vi "Simple Actor Example.vi"() -> ()   [LabVIEW 2012]
uses:
  <vilib>/ActorFramework/Message Enqueuer/Message Enqueuer.lvclass
  <vilib>/ActorFramework/LastAck/Last Ack.lvclass
  <vilib>/ActorFramework/Message Queue/Message Queue.lvclass/Message Queue.ctl
  <vilib>/ActorFramework/Message Dequeuer/Message Dequeuer.lvclass/Message Dequeuer.ctl
  Simple Actor/Simple Actor.lvclass
  <vilib>/ActorFramework/LastAck/Last Ack.lvclass/Last Ack.ctl
  Simple Actor/Simple Actor.lvclass/Simple Actor.ctl
  <vilib>/ActorFramework/Message Enqueuer/Message Enqueuer.lvclass/Message Enqueuer.ctl
  <vilib>/ActorFramework/Message Enqueuer/Enqueue.vi
  <vilib>/ActorFramework/Message Priority Queue/Priority Dequeue.vi
  <vilib>/ActorFramework/Message Priority Queue/Priority Enqueue.vi
  <vilib>/ActorFramework/Stop Msg/Stop Msg.lvclass
  Simple Actor Messages/Zero Msg/Zero Msg.lvclass
  <vilib>/ActorFramework/Actor/Actor.lvclass
  <vilib>/ActorFramework/Message Queue/Message Queue.lvclass
  <vilib>/ActorFramework/Message Dequeuer/Message Dequeuer.lvclass
panel:
  in  "Target Actor":u16(ring) items=["0", "2"]
  in  "Synch":bool
  in  "Process Stop Button":bool
  in  "Refresh Button":bool
  in  "New Button":bool
  in  "stop":bool
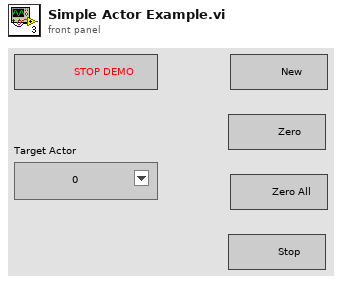
[diagram p1: front panel]
types:
  T1 = enum8{"Enabled", "Disabled", "Disabled and Grayed Out"}
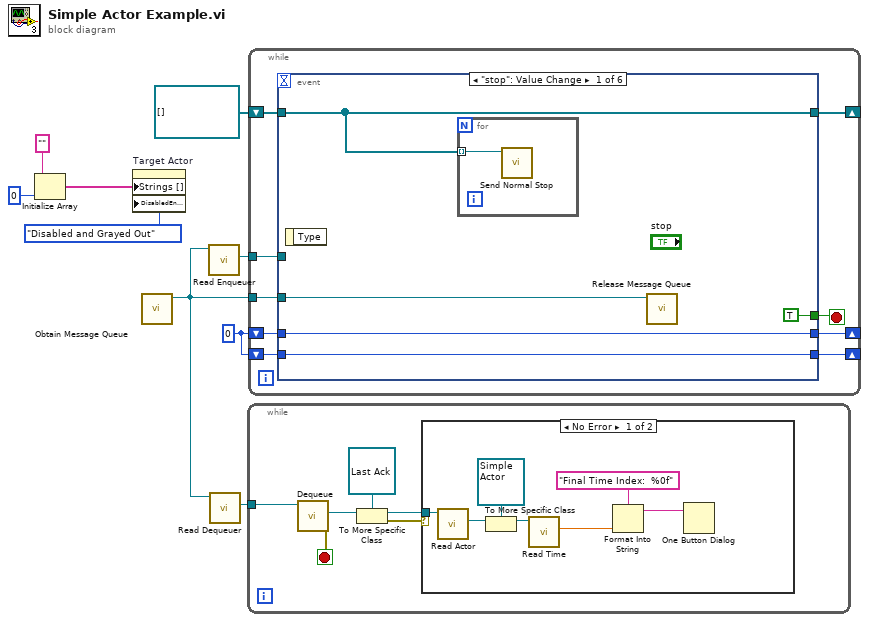
[diagram p0: block diagram]
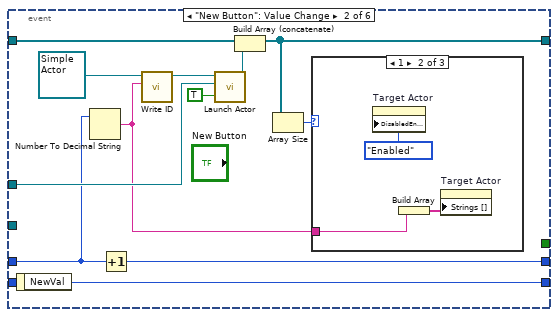
[diagram p3: hidden frame]
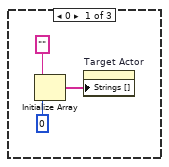
[diagram p4: hidden frame]
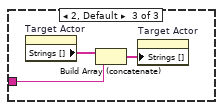
[diagram p5: hidden frame]
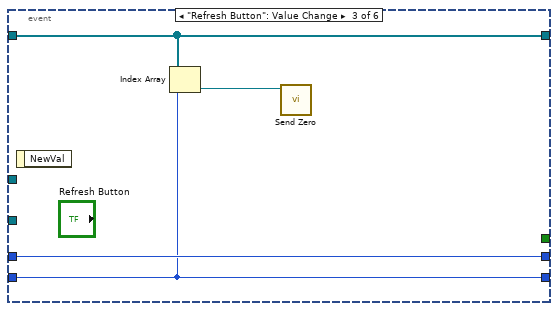
[diagram p6: hidden frame]
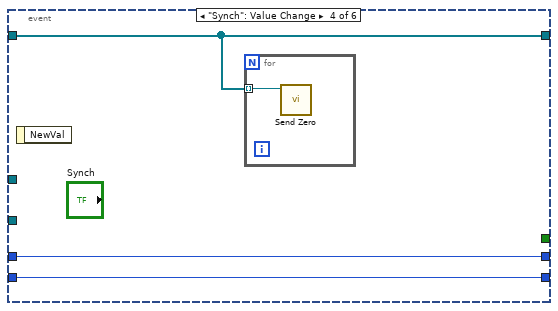
[diagram p7: hidden frame]
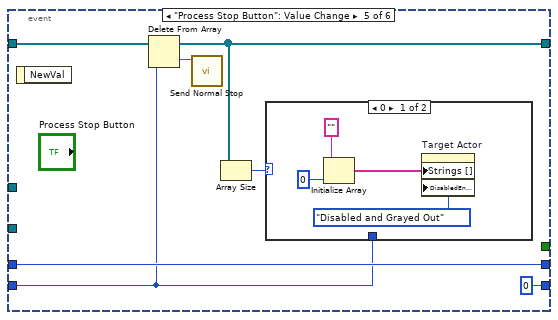
[diagram p8: hidden frame]
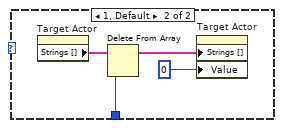
[diagram p9: hidden frame]
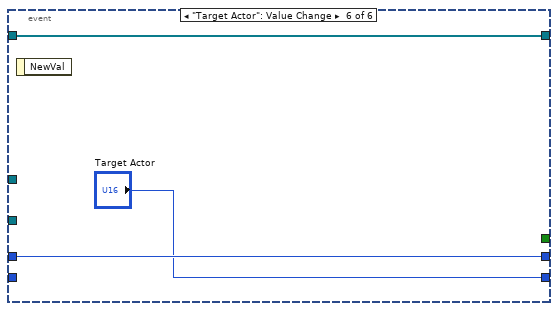
[diagram p10: hidden frame]
diagram:
  w5 = 0
  n1 = Initialize Array("", 0 ("dimension size")) -> (w4:string[])
  n2 = property on="Target Actor" class="Ring (strict)"("Strings []"=w4, "DisabledEnum"=T1."Disabled and Grayed Out" ("Disabled")) -> ()  [unwired: 2 in, 2 out]
  n3 = call <vilib>:"Obtain Message Queue.vi"() -> ("Message Queue"=w7:refnum<class "Message Queue.lvclass">)  [unwired: 10 in, 1 out]
  n4 = call <vilib>:"Read Enqueuer.vi"("Message Queue"=w7) -> ("Message Enqueuer"=w9:refnum<class "Message Enqueuer.lvclass">)  [unwired: 10 in]
  n5 = call <vilib>:"Read Dequeuer.vi"("Message Queue"=w7) -> ("Message Dequeuer"=w6:refnum<class "Message Dequeuer.lvclass">)  [unwired: 10 in]
  n6 = while {
    tunnel: w6 -> [w15]
    stop <- w14 stop-if-true
    n7 = call <vilib>:"Dequeue.vi"("Message Dequeuer in"=w15) -> ("error out"=w14:errorcluster, "Message"=w13:refnum<class "Message.lvclass">)  [unwired: 7 in, 2 out]
    n8 = To More Specific Class(target class=refnum<class "Last Ack.lvclass"> refnum ("Actor Framework.lvlib:Last Ack"), reference=w13) -> (specific class reference=w11:refnum<class "Last Ack.lvclass">, error out=w10:errorcluster)  [unwired: 1 in]
    n9 = case shown="No Error" w10 {
      tunnel: w11 -> [w22 _]
      frame No Error {
        n10 = call <vilib>:"Read Actor.vi"("Last Ack"=w22) -> ("Actor"=w21:refnum<class "Actor.lvclass">)  [unwired: 10 in]
        n11 = To More Specific Class(target class=refnum<class "Simple Actor.lvclass"> refnum ("Simple Actor.lvclass"), reference=w21) -> (specific class reference=w19:refnum<class "Simple Actor.lvclass">)  [unwired: 1 in, 1 out]
        n12 = call "Read Time.vi"("Simple Actor in"=w19) -> ("Time"=w18:dbl)  [unwired: 9 in, 1 out]
        n13 = Format Into String(format string="Final Time Index:  %0f", w18) -> (resulting string=w16:string)  [unwired: 2 in, 1 out]
        n14 = One Button Dialog(message=w16) -> ()  [unwired: 1 in, 1 out]
      }
      frame Error {
      }
    }
  }
  n15 = while {
    tunnel: w7 -> [w31]
    shift-right: [w27] -> _
    shift-left: refnum<class "Message Enqueuer.lvclass">[] [] -> [w29]
    tunnel: w9 -> [w28]
    shift-right: [w25] -> _
    shift-left: w5 -> [w26]
    shift-right: [w24] -> _
    shift-left: w5 -> [w23]
    stop <- w30 stop-if-true
    n16 = event shown="[0] \"stop\": Value Change" {
      selector: _ -> [_ _ _ _ _ _]
      dyn-events: _ -> [_ _ _ _ _ _]
      timeout: _ -> [_ _ _ _ _ _]
      tunnel: w31 -> [w36 _ _ _ _ _]
      tunnel: [TRUE _ _ _ _ _] -> w30
      tunnel: w29 -> [w34 w47 w62 w65 w73 w82]
      tunnel: w28 -> [_ w48 _ _ _ _]
      tunnel: [w34 w45 w62 w65 w71 w82] -> w27
      tunnel: w26 -> [w33 w41 w60 w64 w69 w84]
      tunnel: [w33 w40 w60 w64 w69 w84] -> w25
      tunnel: [w32 w39 w59 w63 0 ("Target Actor") "Target Actor"] -> w24
      tunnel: w23 -> [w32 w39 w59 w63 w68 _]
      event "stop": Value Change {
        n17 = event-data() -> ()  [unwired: 1 in, 1 out]
        n18 = for {
          tunnel: w34 -> [w37] mode=indexing
          n19 = call <vilib>:"Send Normal Stop.vi"("Message Enqueuer"=w37) -> ()  [unwired: 10 in, 1 out]
        }
        n20 = call <vilib>:"Release Message Queue.vi"("Message Queue"=w36) -> ()  [unwired: 9 in, 2 out]
      }
      event "New Button": Value Change {
        n21 = event-data() -> ()  [unwired: 1 in, 1 out]
        n22 = Number To Decimal String(number=w41) -> (decimal integer string=w38:string)  [unwired: 1 in]
        n23 = Increment(x=w41) -> (x+1=w40:i32)
        n24 = call "Write ID.vi"("ID"=w38, "Simple Actor in"=refnum<class "Simple Actor.lvclass"> refnum ("Simple Actor.lvclass")) -> ("Simple Actor out"=w42:refnum<class "Simple Actor.lvclass">)  [unwired: 9 in]
        n25 = call <vilib>:"Launch Actor.vi"("Open Actor Core front panel? (F)"=TRUE, "Actor-to-Caller Enqueuer"=w48, "Actor"=w42) -> ("Caller-To-Actor Enqueuer"=w46:refnum<class "Message Enqueuer.lvclass">)  [unwired: 7 in, 1 out]
        n26 = Build Array (concatenate)(w47, w46) -> (w45:refnum<class "Message Enqueuer.lvclass">[])
        n27 = Array Size(array=w45) -> (size(s)=w44:i32)
        n28 = case shown="1" w44 {
          tunnel: w38 -> [_ w53 w56]
          frame 0 {
            n29 = Initialize Array("", 0 ("dimension size")) -> (w51:string[])
            n30 = property on="Target Actor" class="Ring (strict)"("Strings []"=w51) -> ()  [unwired: 2 in, 2 out]
          }
          frame 1 {
            n31 = property on="Target Actor" class="Ring (strict)"("DisabledEnum"=T1."Enabled" ("Disabled")) -> ()  [unwired: 2 in, 2 out]
            n32 = Build Array(w53) -> (w54:string[])
            n33 = property on="Target Actor" class="Ring (strict)"("Strings []"=w54) -> ()  [unwired: 2 in, 2 out]
          }
          frame 2, Default {
            n34 = property on="Target Actor" class="Ring (strict)"() -> ("Strings []"=w58:string[])  [unwired: 2 in, 2 out]
            n35 = Build Array (concatenate)(w58, w56) -> (w57:string[])
            n36 = property on="Target Actor" class="Ring (strict)"("Strings []"=w57) -> ()  [unwired: 2 in, 2 out]
          }
        }
      }
      event "Refresh Button": Value Change {
        n37 = event-data() -> ()  [unwired: 1 in, 1 out]
        n38 = Index Array(array=w62, index=w59) -> (element=w61:refnum<class "Message Enqueuer.lvclass">)
        n39 = call "Send Zero.vi"("Message Enqueuer"=w61) -> ()  [unwired: 9 in, 2 out]
      }
      event "Synch": Value Change {
        n40 = event-data() -> ()  [unwired: 1 in, 1 out]
        n41 = for {
          tunnel: w65 -> [w66] mode=indexing
          n42 = call "Send Zero.vi"("Message Enqueuer"=w66) -> ()  [unwired: 9 in, 2 out]
        }
      }
      event "Process Stop Button": Value Change {
        n43 = event-data() -> ()  [unwired: 1 in, 1 out]
        n44 = Delete From Array(array=w73, index=w68) -> (deleted portion=w72:refnum<class "Message Enqueuer.lvclass">, array with subset deleted=w71:refnum<class "Message Enqueuer.lvclass">[])  [unwired: 1 in]
        n45 = call <vilib>:"Send Normal Stop.vi"("Message Enqueuer"=w72) -> ()  [unwired: 10 in, 1 out]
        n46 = Array Size(array=w71) -> (size(s)=w70:i32)
        n47 = case shown="0" w70 {
          tunnel: w68 -> [_ w79]
          frame 0 {
            n48 = Initialize Array("", 0 ("dimension size")) -> (w74:string[])
            n49 = property on="Target Actor" class="Ring (strict)"("Strings []"=w74, "DisabledEnum"=T1."Disabled and Grayed Out" ("Disabled")) -> ()  [unwired: 2 in, 2 out]
          }
          frame 1, Default {
            n50 = property on="Target Actor" class="Ring (strict)"() -> ("Strings []"=w80:string[])  [unwired: 2 in, 2 out]
            n51 = Delete From Array(array=w80, index=w79) -> (array with subset deleted=w81:string[])  [unwired: 1 in, 1 out]
            n52 = property on="Target Actor" class="Ring (strict)"("Strings []"=w81, "Value"=0 ("dimension size")) -> ()  [unwired: 2 in, 2 out]
          }
        }
      }
      event "Target Actor": Value Change {
        n53 = event-data() -> ()  [unwired: 1 in, 1 out]
      }
    }
  }
